vi "Update Digital Pattern Cursor Controls.vi"(8 "error in (no error)":errorcluster, 11 "Page Data in":T1={"SysExp Event"=refnum, "Init done"=FALSE, "Node Ptr"=18446744073709551615, "Ctrl Refs"={"Header"=refnum, "Pattern Plot"=refnum, "Zoom"=refnum, "Select Pattern"=refnum, "Add List"=refnum, "Remove List"=refnum, "Pattern Name"=refnum, "remove_add"=refnum, "remove_remove"=refnum, "add_remove"=refnum, "base_Length"=refnum, "base_teeth"=refnum, "base_Toothwidth"=refnum, "base_Offset"=refnum, "add_Tooth"=refnum, "add_Width"=refnum, "add_Offset"=refnum, "remove_Tooth"=refnum, "remove_Edge"=refnum, "Chart_Position"=refnum, "Chart_Tooth"=refnum, "Chart_Offset"=refnum, "add_add"=refnum, "pattern_remove"=refnum, "pattern_add"=refnum, "FPGA Resource"=refnum}, "SE ref"=refnum, "Patterns"=[], "Sel patterns"=[], "rotations"=0, "Need save"=FALSE, "Rem List"=0, "Add List"=0, "FPGA Resources"=[]} {"Node Ptr" format="%.0x"}) -> (0 "error out":errorcluster)   [LabVIEW 2019, in "Engine Simulation Toolkit System Explorer.lvlib"]
uses:
  Engine Simulation Toolkit System Explorer.lvlib
  Digital Patterns Page Data.ctl
  <vilib>/NI VeriStand/Custom Device API/Custom Device Item Ref.ctl
  Digital Pattern.ctl
  Digital Pattern Base.ctl
  Digital Pattern Remove Edge.ctl
  Digital Pattern Add Pulse.ctl
  <vilib>/NI VeriStand/Custom Device API/Custom Device API.lvlib
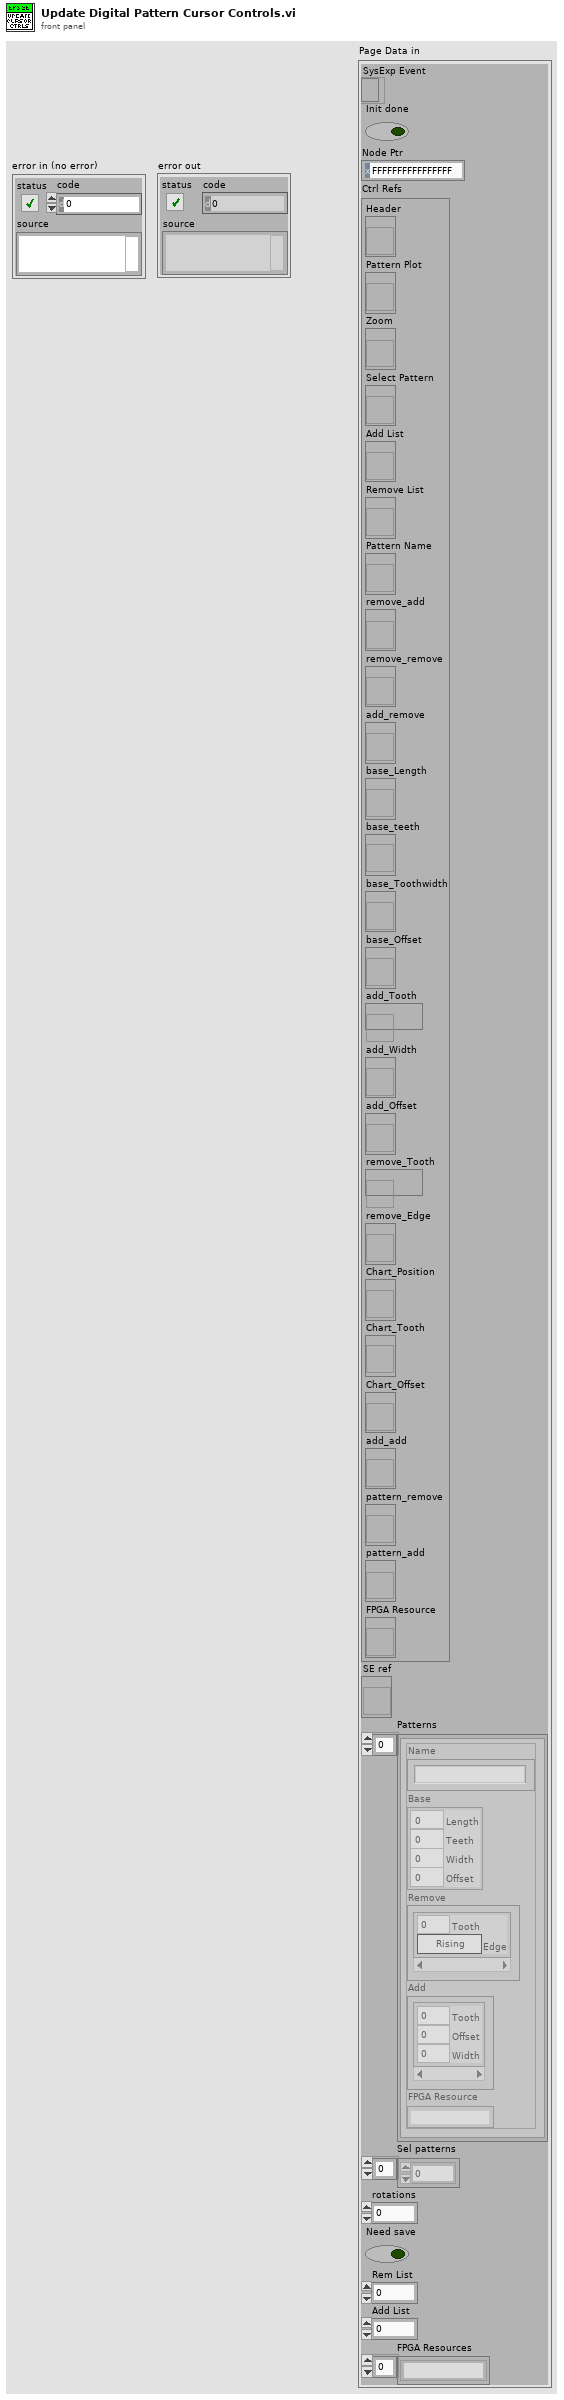
[diagram p1: front panel]
types:
  T1 = typedef "Engine Simulation Toolkit System Explorer.lvlib/Digital Patterns Page Data.ctl" = cluster{"SysExp Event":refnum<event-registration>, "Init done":bool, "Node Ptr":T2, "Ctrl Refs":cluster{"Header":refnum<vi>, "Pattern Plot":refnum<vi>, "Zoom":refnum<vi>, "Select Pattern":refnum<vi>, "Add List":refnum<vi>, "Remove List":refnum<vi>, "Pattern Name":refnum<vi>, "remove_add":refnum<vi>, "remove_remove":refnum<vi>, "add_remove":refnum<vi>, "base_Length":refnum<vi>, "base_teeth":refnum<vi>, "base_Toothwidth":refnum<vi>, "base_Offset":refnum<vi>, "add_Tooth":refnum<vi>, "add_Width":refnum<vi>, "add_Offset":refnum<vi>, "remove_Tooth":refnum<vi>, "remove_Edge":refnum<vi>, "Chart_Position":refnum<vi>, "Chart_Tooth":refnum<vi>, "Chart_Offset":refnum<vi>, "add_add":refnum<vi>, "pattern_remove":refnum<vi>, "pattern_add":refnum<vi>, "FPGA Resource":refnum<vi>}, "SE ref":refnum<vi>, "Patterns":T3[], "Sel patterns":i32[], "rotations":u16, "Need save":bool, "Rem List":i32, "Add List":i32, "FPGA Resources":string[]}
  T2 = typedef "Custom Device API.lvlib/Custom Device Item Ref.ctl" = u64
  T3 = typedef "Engine Simulation Toolkit System Explorer.lvlib/Digital Pattern.ctl" = cluster{"Name":string, "Base":T4, "Remove":T5[], "Add":T6[], "FPGA Resource":string}
  T4 = typedef "Engine Simulation Toolkit System Explorer.lvlib/Digital Pattern Base.ctl" = cluster{"Length":dbl, "Teeth":u16, "Width":dbl, "Offset":dbl}
  T5 = typedef "Engine Simulation Toolkit System Explorer.lvlib/Digital Pattern Remove Edge.ctl" = cluster{"Tooth":u16, "Edge":bool}
  T6 = typedef "Engine Simulation Toolkit System Explorer.lvlib/Digital Pattern Add Pulse.ctl" = cluster{"Tooth":u16, "Offset":dbl, "Width":dbl}
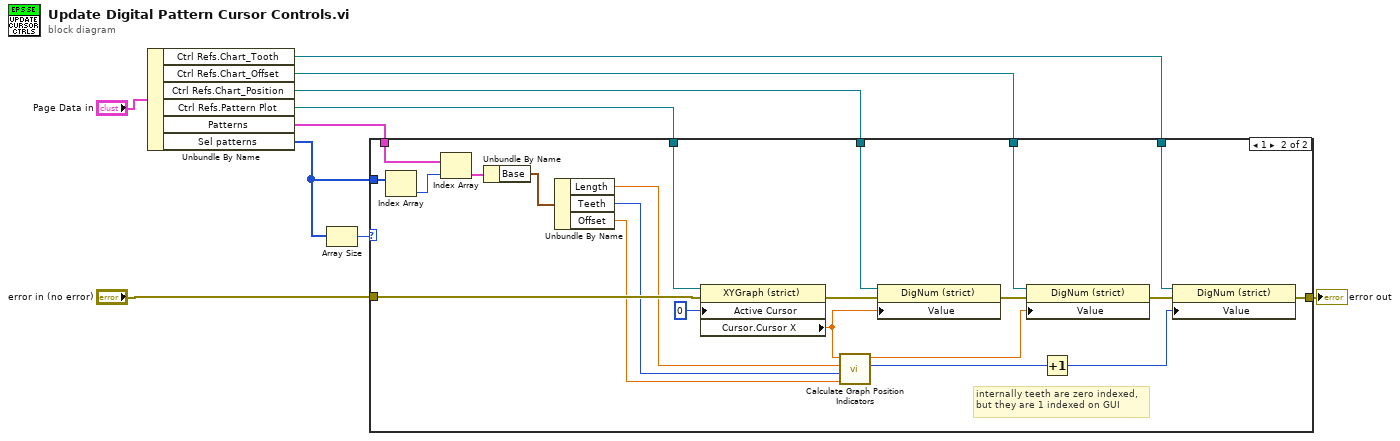
[diagram p0: block diagram]
diagram:
  n1 = Unbundle By Name("Page Data in") -> ("Ctrl Refs.Chart_Tooth"=w5:refnum<vi>, "Ctrl Refs.Chart_Offset"=w6:refnum<vi>, "Ctrl Refs.Chart_Position"=w7:refnum<vi>, "Ctrl Refs.Pattern Plot"=w8:refnum<vi>, "Patterns"=w3:T3[], "Sel patterns"=w2:i32[])
  n2 = Array Size(array=w2) -> (size(s)=w1:i32)
  n3 = case shown="1" w1 {
    tunnel: "error in (no error)" -> [w11 w30]
    tunnel: w8 -> [_ w29]
    tunnel: w7 -> [_ w21]
    tunnel: w6 -> [_ w20]
    tunnel: w5 -> [_ w19]
    tunnel: [w11 w16] -> w4
    tunnel: w3 -> [_ w14]
    tunnel: w2 -> [_ w12]
    frame Default {
    }
    frame 1 {
      # "internally teeth are zero indexed, but they are 1 indexed on GUI"
      n4 = Index Array(array=w12) -> (element=w33:i32)  [unwired: 1 in]
      n5 = Index Array(array=w14, index=w33) -> (element=w32:T3)
      n6 = Unbundle By Name(w32) -> ("Base"=w31:T4)
      n7 = Unbundle By Name(w31) -> ("Length"=w25:dbl, "Teeth"=w24:u16, "Offset"=w15:dbl)
      n8 = property on="Property Node" class="XYGraph (strict)"(reference=w29, error in=w30, "Active Cursor"=u32 0) -> (error out=w27:errorcluster, "Cursor.Cursor X"=w28:dbl)  [unwired: 1 out]
      n9 = call "Calculate Graph Position Indicators.vi"("Pattern offset"=w15, "Pattern teeth"=w24, "Pattern length"=w25, "Cursor position"=w28) -> ("Tooth"=w17:u16, "Offset"=w18:dbl)  [unwired: 6 in]
      n10 = property on="Property Node" class="DigNum (strict)"(reference=w21, error in=w27, "Value"=w28) -> (error out=w22:errorcluster)  [unwired: 1 out]
      n11 = property on="Property Node" class="DigNum (strict)"(reference=w20, error in=w22, "Value"=w18) -> (error out=w23:errorcluster)  [unwired: 1 out]
      n12 = Increment(x=w17) -> (x+1=w13:u16)
      n13 = property on="Property Node" class="DigNum (strict)"(reference=w19, error in=w23, "Value"=w13) -> (error out=w16:errorcluster)  [unwired: 1 out]
    }
  }
  "error out" <- w4
